vi "remote.Set NVMEM Bytes.vi"(0 "SLSC Remote in":refnum<class "SLSC Interface.lvclass">, 5 "NVMEM area":refnum<k21>="$DefaultNVMEMAreas", 7 "data address":u32 format="%.0x", 9 "data":u8[](array[numeric]) format="%.0x", 11 "error in (no error)":errorcluster) -> (4 "SLSC Remote out":refnum<class "SLSC Interface.lvclass">, 6 "NVMEM area out":refnum<k21>, 8 "next data address":u32 format="%.0x", 15 "error out":errorcluster)   [LabVIEW 2016, in "SLSC Interface.lvclass"]
uses:
  SLSC Interface Class/SLSC Interface.lvclass
  SLSC Interface Class/SLSC Interface.lvclass/SLSC Interface.ctl
  SLSC Interface Class/Read client handle.vi
  SLSC Interface Class/Read URL.vi
  <vilib>/NI/JSON Support for LabVIEW/JSON Data Classes/JSON Object/JSON Object.lvclass
  C:/Program Files (x86)/National Instruments/LabVIEW 2016/vi.lib/NI/JSON Support for LabVIEW/JSON Data Classes/JSON Datatype/JSON Null.lvclass
  SLSC Interface Class/Read session.vi
  <vilib>/NI/JSON Support for LabVIEW/JSON Data Classes/JSON Object/New JSON Object (Empty).vi
  <vilib>/NI/JSON Support for LabVIEW/JSON Data Classes/JSON Object/Insert Key Value Pair (Single String).vi
  <vilib>/NI/JSON Support for LabVIEW/JSON Data Classes/JSON Object/Insert Key Value Pair (Single Numeric).vi
  <vilib>/NI/NI JSONRPC Server Framework/Classes/Server/Format Client Request (Auto-Increment).vi
  <vilib>/httpClient/POSTBuffer.vi
  <vilib>/NI/NI JSONRPC Server Framework/Classes/Server/Parse Response (Object).vi
  <vilib>/NI/JSON Support for LabVIEW/JSON Data Classes/JSON Object/Get Value (Numeric Value).vi
  <vilib>/NI/NI JSONRPC Server Framework/Classes/Server/JSONRPC Server.lvclass
  <vilib>/httpClient/LabVIEWHTTPClient.lvlib
  <vilib>/NI/JSON Support for LabVIEW/JSON Data Classes/JSON Helper/JSON Helper.lvclass
  C:/Program Files (x86)/National Instruments/LabVIEW 2016/vi.lib/NI/JSON Support for LabVIEW/JSON Data Classes/JSON Structured Type/JSON Structure.lvclass
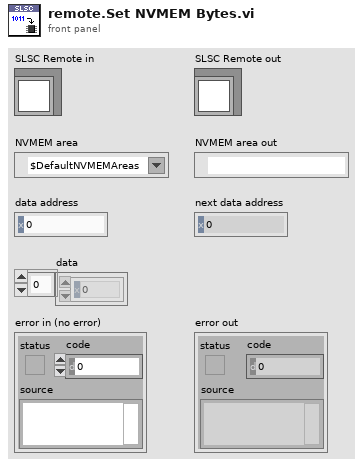
[diagram p1: front panel]
types:
  T1 = typedef "LabVIEWHTTPClient.lvlib/ClientHandle.ctl" = refnum<k1>
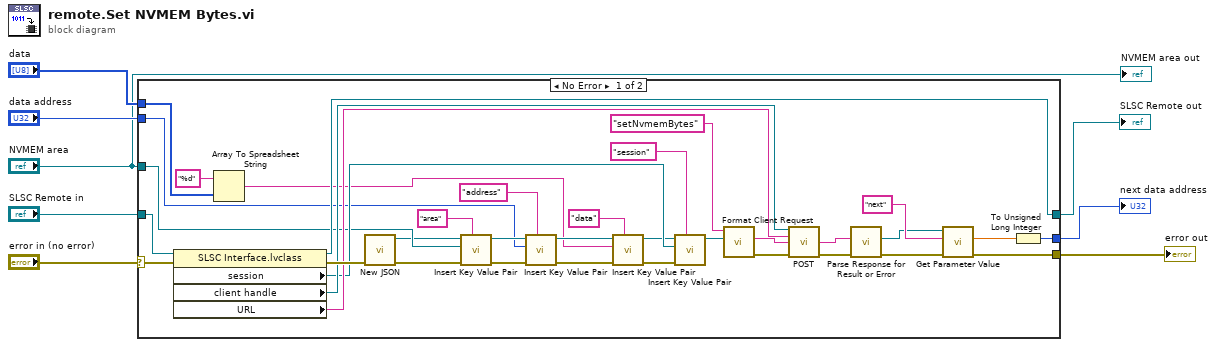
[diagram p0: block diagram]
diagram:
  n1 = case shown="No Error" "error in (no error)" {
    selector: "error in (no error)" -> [w43 w46]
    tunnel: "NVMEM area" -> [w22 _]
    tunnel: [w44 w45] -> w2
    tunnel: "data address" -> [w13 _]
    tunnel: "data" -> [w11 _]
    tunnel: [w27 w46] -> w1
    tunnel: "SLSC Remote in" -> [w29 w45]
    tunnel: [w25 _] -> w8
    frame No Error {
      n2 = property class="SLSC Interface.lvclass"(reference=w29, error in=w43) -> (reference out=w44:refnum<class "SLSC Interface.lvclass">, error out=w42:errorcluster, "session"=w23:refnum<k21>, "client handle"=w35:T1, "URL"=w34:string)
      n3 = Array To Spreadsheet String(array=w11, 3:"%d" ("format string")) -> (spreadsheet string=w10:string)  [unwired: 1 in]
      n4 = call-poly <vilib>:"New JSON.vi"("error in (no error)"=w42) -> ("error out"=w41:errorcluster, "JSON Object out"=w17:refnum<class "JSON Object.lvclass">)  [unwired: 9 in]
      n5 = call-poly <vilib>:"Insert Key Value Pair.vi"("key"="area" ("Name"), "error in (no error)"=w41, "value"=w22, "JSON Object in"=w17) -> ("error out"=w40:errorcluster, "JSON Object out"=w16:refnum<class "JSON Object.lvclass">)  [unwired: 5 in, 1 out]
      n6 = call-poly <vilib>:"Insert Key Value Pair.vi"("key"="address" ("Name"), "error in (no error)"=w40, "value"=w13, "JSON Object in"=w16) -> ("error out"=w37:errorcluster, "JSON Object out"=w15:refnum<class "JSON Object.lvclass">)  [unwired: 5 in, 1 out]
      n7 = call-poly <vilib>:"Insert Key Value Pair.vi"("key"="data" ("String"), "error in (no error)"=w37, "value"=w10, "JSON Object in"=w15) -> ("error out"=w36:errorcluster, "JSON Object out"=w14:refnum<class "JSON Object.lvclass">)  [unwired: 5 in, 1 out]
      n8 = call-poly <vilib>:"Insert Key Value Pair.vi"("key"="session" ("Name"), "error in (no error)"=w36, "value"=w23, "JSON Object in"=w14) -> ("JSON Object out"=w30:refnum<class "JSON Object.lvclass">)  [unwired: 5 in, 2 out]
      n9 = call-poly <vilib>:"Format Client Request.vi"("JSON in"=w30, "method"="setNvmemBytes") -> ("error out"=w33:errorcluster, "Request String"=w38:string)  [unwired: 8 in]
      n10 = call-poly <vilib>:"POST.vi"("client handle"=w35, "url"=w34, "buffer"=w38, "error in (no error)"=w33) -> ("body"=w32:string, "error out"=w31:errorcluster)  [unwired: 8 in, 2 out]
      n11 = call-poly <vilib>:"Parse Response for Result or Error.vi"("error in"=w31, "Response String In"=w32) -> ("error out"=w24:errorcluster, "JSON Array"=w9:refnum<class "JSON Object.lvclass">)  [unwired: 7 in, 1 out]
      n12 = call-poly <vilib>:"Get Parameter Value.vi"("error in (no error)"=w24, "key"="next" ("Parameter Name"), "JSON Object in"=w9) -> ("error out"=w27:errorcluster, "value"=w26:dbl)  [unwired: 7 in]
      n13 = To Unsigned Long Integer(number=w26) -> (unsigned 32bit integer=w25:u32)
    }
    frame Error {
    }
  }
  "error out" <- w1
  "SLSC Remote out" <- w2
  "next data address" <- w8
  "NVMEM area out" <- "NVMEM area"
